vi "UNDTStringToCluster(SubVI).vi"(5 "OptionPACK5":T1={"MagicWordStr"="xV4\u0012", "Header size"=56, "Проверка CRC8"=TRUE, "Проверка конца пакета"=FALSE, "GainCompens"=FALSE, "Неотбрасывать BadEnd пакеты"=TRUE, "Неотбрасывать BadCRC пакеты"=TRUE, "Привести к 1"=FALSE, "GainCoef"=FALSE, "K_scale"=0.0, "ScaleOrdinate"=enum."Проценты"}, 8 "error in":errorcluster, 10 "offset":i32, 11 "data_in":string) -> (0 "error out":errorcluster, 2 "CRC8Good":bool=TRUE, 3 "UNDT_Cluster 3":T2 {"Gain Coeff" format="%#_6e"; "Reserve 1" format="%02x"; "Mux TX/RX" format="%02x"; "ScanDelay" format="%02x"; "PacketCounter" format="%08x"; "SamplingInterval" format="%#_6e"; "Lose Packet" format="%08x"; "EncodersParam2" format="%016x"; "EncodersParam1" format="%016x"; "CRC 8" format="%02x"; "N chanel" format="%02x"; "N tick" format="%02x"; "Ncycle" format="%04x"; "FrameFormatVersion" format="%02x"; "MagicWord" format="%.0x"}, 4 "SizeToSmall":bool)   [LabVIEW 2017]
uses:
  Control_EU/UNDT_ClusterPackRevers (Type).ctl
  Control_EU/OptionPACK5.ctl
panel:
  out "substring":string
  out "length":i32
  out "CRC8_CCITT":u8=139 format="%1x"
  out "CRC8":u8=139 format="%02x"
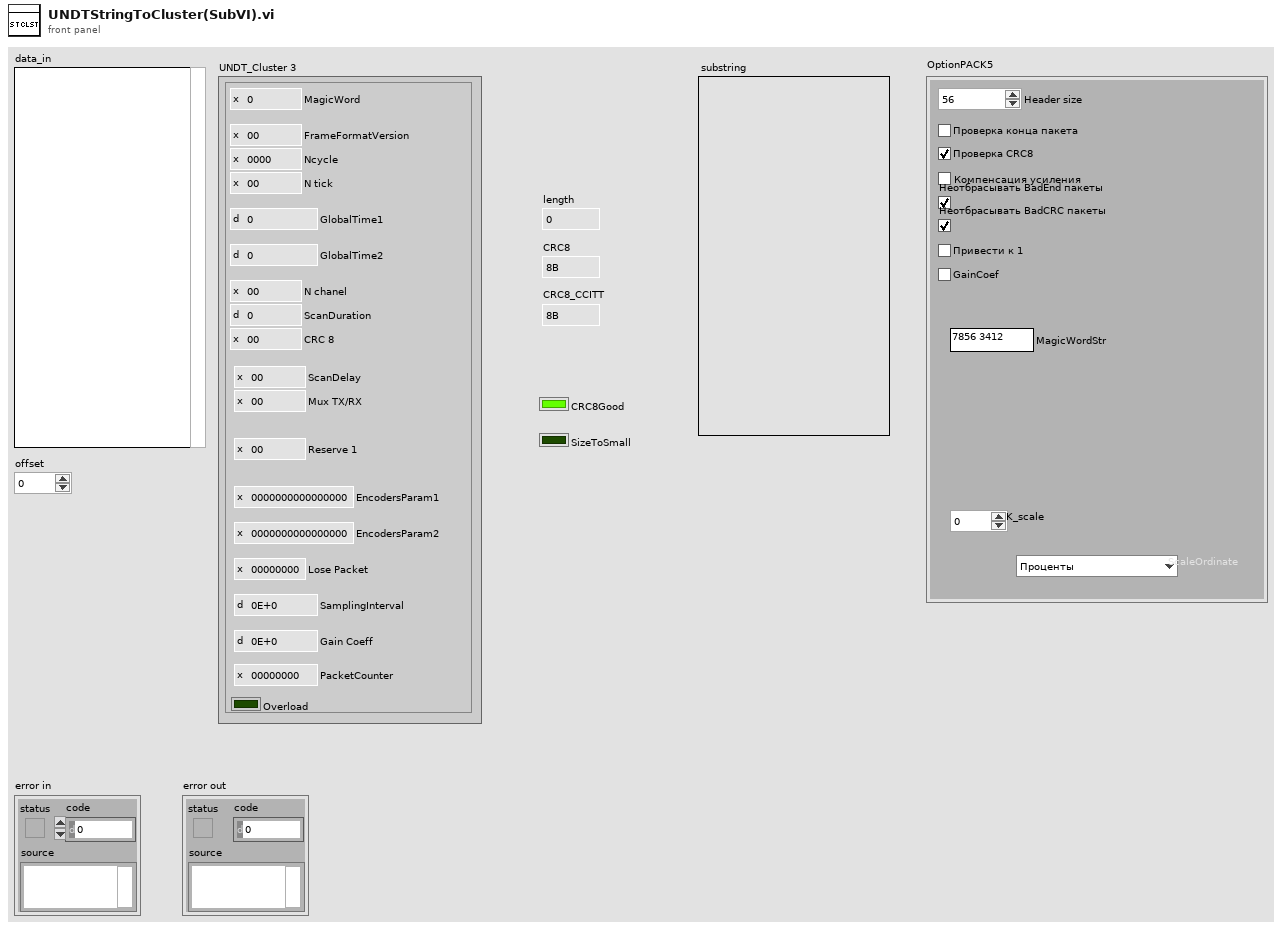
[diagram p1: front panel]
types:
  T1 = typedef "OptionPACK5.ctl" = cluster{"MagicWordStr":string, "Header size":u32, "Проверка CRC8":bool, "Проверка конца пакета":bool, "GainCompens":bool, "Неотбрасывать BadEnd пакеты":bool, "Неотбрасывать BadCRC пакеты":bool, "Привести к 1":bool, "GainCoef":bool, "K_scale":dbl, "ScaleOrdinate":enum16{"Отсчеты АЦП (±32767)", "Проценты", "Вольты", "дБмкВ (отн. 1 мкВ)", "Отсчеты АЦП (±1)"}}
  T2 = typedef "UNDT_ClusterPackRevers (Type).ctl" = cluster{"PacketCounter":u32, "Gain Coeff":sgl, "SamplingInterval":sgl, "Lose Packet":u32, "EncodersParam2":u64, "EncodersParam1":u64, "Reserve 1":u8, "Mux TX/RX":u8, "ScanDelay":u16, "CRC 8":u8, "ScanDuration":u16, "N chanel":u8, "GlobalTime2":u32, "GlobalTime1":u32, "N tick":u8, "Ncycle":u16, "FrameFormatVersion":u8, "MagicWord":u32, "Overload":bool}
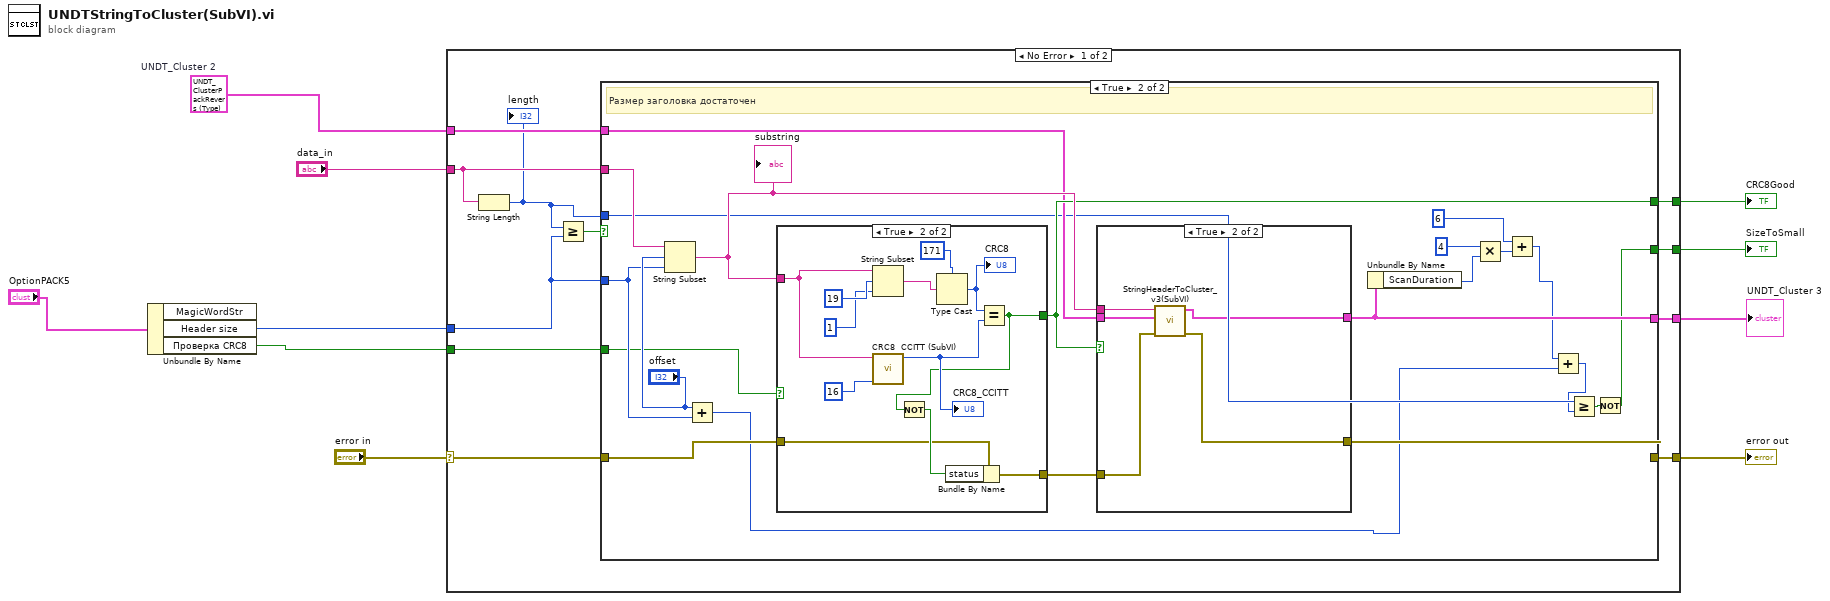
[diagram p0: block diagram]
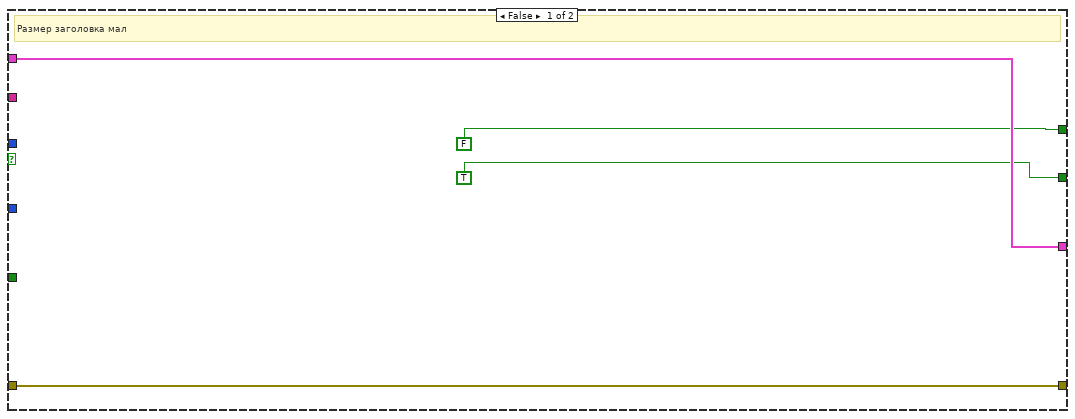
[diagram p2: hidden frame]
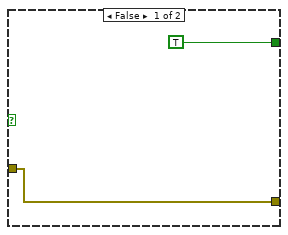
[diagram p4: hidden frame]
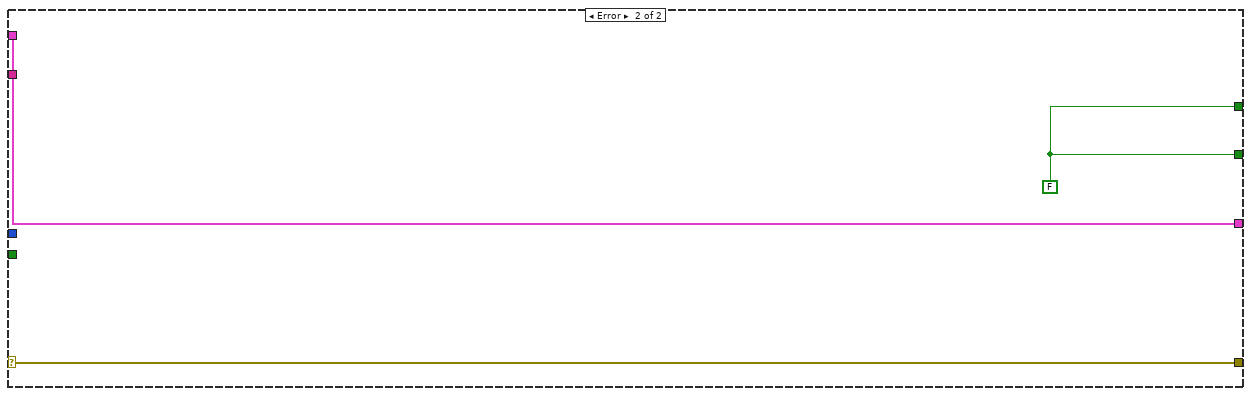
[diagram p5: hidden frame]
diagram:
  w6 = T2 {"PacketCounter"=0, "Gain Coeff"=0.0, "SamplingInterval"=0.0, "Lose Packet"=0, "EncodersParam2"=0, "EncodersParam1"=0, "Reserve 1"=0, "Mux TX/RX"=0, "ScanDelay"=0, "CRC 8"=0, "ScanDuration"=0, "N chanel"=0, "GlobalTime2"=0, "GlobalTime1"=0, "N tick"=0, "Ncycle"=0, "FrameFormatVersion"=0, "MagicWord"=0, "Overload"=FALSE}  # UNDT_Cluster 2
  n1 = Unbundle By Name("OptionPACK5") -> ("Header size"=w2:u32, "Проверка CRC8"=w1:bool)  [unwired: 1 out]
  n2 = case shown="No Error" "error in" {
    selector: "error in" -> [w17 w69]
    tunnel: [w21 w68] -> w10
    tunnel: w6 -> [w14 w70]
    tunnel: [w20 w70] -> w5
    tunnel: "data_in" -> [w19 _]
    tunnel: [w16 w69] -> w9
    tunnel: [w15 w68] -> w7
    tunnel: w2 -> [w12 _]
    tunnel: w1 -> [w11 _]
    frame No Error {
      n3 = String Length(string=w19) -> (length=w13:i32)
      "length" <- w13
      n4 = Greater Or Equal?(x=w13, y=w12) -> (x >= y?=w18:bool)
      n5 = case shown="True" w18 {
        tunnel: [FALSE w45] -> w21
        tunnel: w14 -> [w25 w40]
        tunnel: [w25 w39] -> w20
        tunnel: w19 -> [_ w41]
        tunnel: w12 -> [_ w28]
        tunnel: w17 -> [w23 w44]
        tunnel: [w23 w43] -> w16
        tunnel: [TRUE w36] -> w15
        tunnel: w13 -> [_ w38]
        tunnel: w11 -> [_ w26]
        frame False {
          # "Размер заголовка мал"
        }
        frame True {
          # "Размер заголовка достаточен"
          n6 = String Subset(string=w41, offset (0)="offset", length (rest)=w28) -> (substring=w46:string)
          "substring" <- w46
          n7 = Add(x="offset", y=w28) -> (x+y=w27:u32)
          n8 = case shown="True" w26 {
            tunnel: w46 -> [_ w59]
            tunnel: [TRUE w65] -> w45
            tunnel: w44 -> [w54 w63]
            tunnel: [w54 w62] -> w42
            frame False {
            }
            frame True {
              n9 = String Subset(string=w59, offset (0)=19, length (rest)=1 ("length (rest)")) -> (substring=w58:string)
              n10 = call "CRC8  CCITT (SubVI).vi"("wLength"=16 ("length (rest)"), "string in"=w59) -> ("CRC8_CCITT"=w66:u8)  [unwired: 9 in]
              "CRC8_CCITT" <- w66
              n11 = Type Cast(type=u8 171 ("CRC8_CCITT"), x=w58) -> (*(type *) &x=w57:u8)
              "CRC8" <- w57
              n12 = Equal?(x=w57, y=w66) -> (x = y?=w65:bool)
              n13 = Not(x=w65) -> (.not. x?=w64:bool)
              n14 = Bundle By Name(cluster=w63, "status"=w64) -> (w62:errorcluster)
            }
          }
          n15 = case shown="True" w45 {
            tunnel: w40 -> [w48 w50]
            tunnel: w46 -> [_ w53]
            tunnel: [w48 w49] -> w39
            tunnel: [w47 w51] -> w43
            tunnel: w42 -> [w47 w52]
            frame False {
            }
            frame True {
              n16 = call "StringHeaderToCluster_v3(SubVI).vi"("error in"=w52, "UNDT_Cluster 2"=w50, "data_in 2"=w53) -> ("error out"=w51:errorcluster, "UNDT_Cluster"=w49:T2)  [unwired: 7 in]
            }
          }
          n17 = Unbundle By Name(w39) -> ("ScanDuration"=w34:u16)
          n18 = Multiply(x=u16 4, y=w34) -> (x*y=w32:u16)
          n19 = Add(x=u16 6, y=w32) -> (x+y=w30:u16)
          n20 = Add(x=w30, y=w27) -> (x+y=w37:u32)
          n21 = Greater Or Equal?(x=w38, y=w37) -> (x >= y?=w35:bool)
          n22 = Not(x=w35) -> (.not. x?=w36:bool)
        }
      }
    }
    frame Error {
      w68 = FALSE
    }
  }
  "CRC8Good" <- w10
  "error out" <- w9
  "SizeToSmall" <- w7
  "UNDT_Cluster 3" <- w5
